vi "Test.vi"() -> ()   [LabVIEW 2014]
uses:
  TypeDefs/TriangleFace.ctl
  TypeDefs/Point3D.ctl
  C:/Users/guss2/Documents/CodeBlocksTest/DLL/bin/Debug/DLL.dll
panel:
  in  "zStart":sgl
  in  "List/Poly":bool
  in  "Layer":i32
  out "XY Graph":cluster{cluster{"X":sgl, "Y":sgl}[]}[](graph)
  out "Length":i32
  out "Triangles":T1[](array[typedef])
  in  "STL Path":path=path "D:/Data/Git/LVslicer/STL2/cone.stl"
  out "NumIntersect":i64
  out "edgeLen":i32[](array[numeric])
  out "List":T3(array[cluster])
  in  "Thick":sgl=0.321
  in  "NumSlices":i32=3
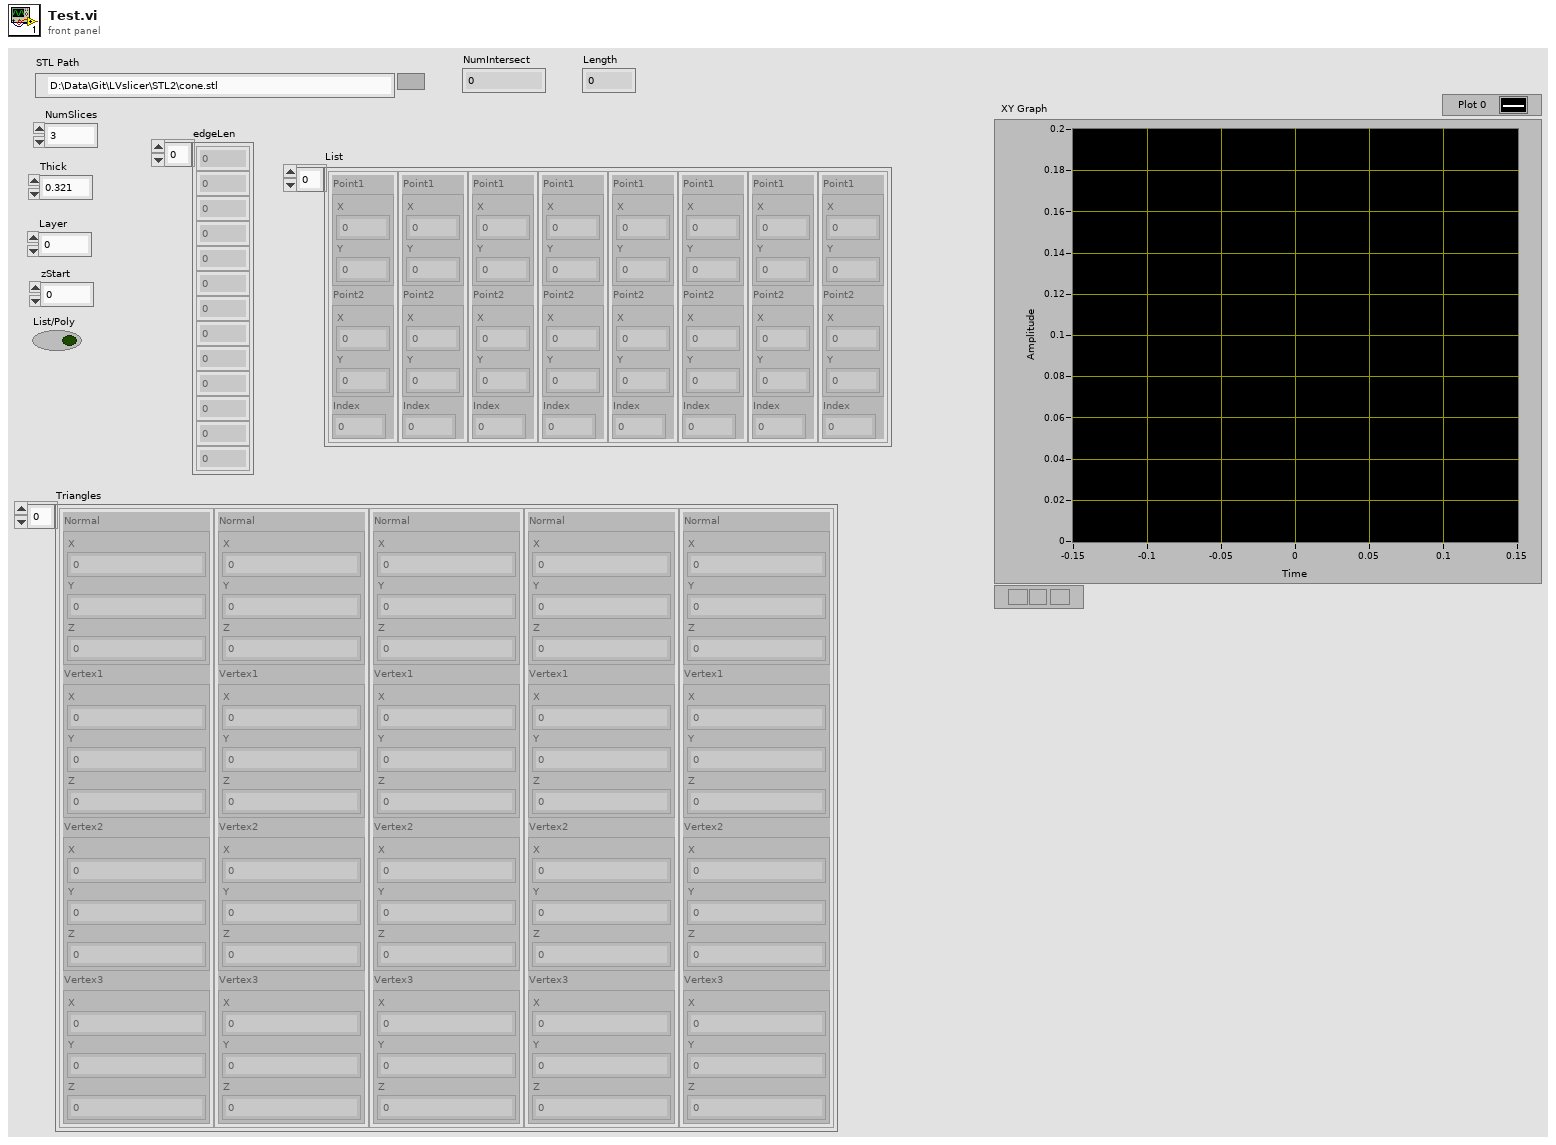
[diagram p1: front panel]
types:
  T1 = typedef "TriangleFace.ctl" = cluster{"Normal":T2, "Vertex1":T2, "Vertex2":T2, "Vertex3":T2}
  T2 = typedef "Point3D.ctl" = cluster{"X":sgl, "Y":sgl, "Z":sgl}
  T3 = cluster{"Point1":cluster{"X":sgl, "Y":sgl}, "Point2":cluster{"X":sgl, "Y":sgl}, "Index":i32}[]
  T4 = cluster{"Point1":cluster{"X":sgl, "Y":sgl}, "Point2":cluster{"X":sgl, "Y":sgl}, "Index":i32}
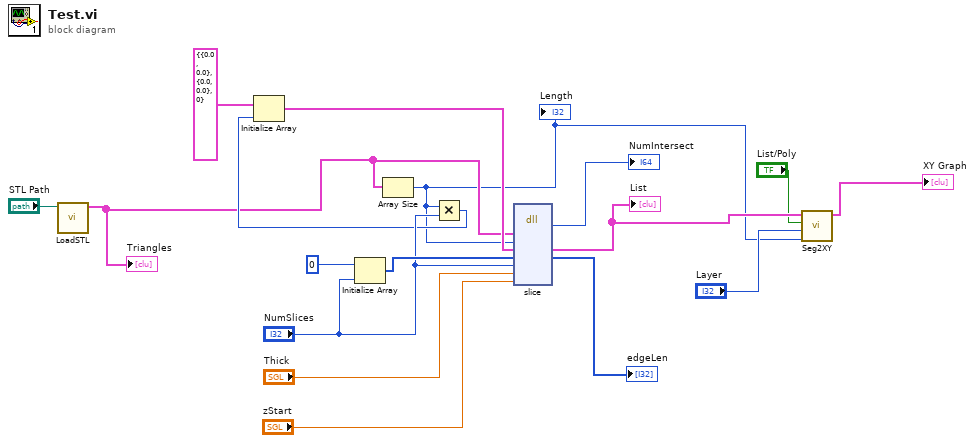
[diagram p0: block diagram]
diagram:
  n1 = call "LoadSTL.vi"("STL Path"="STL Path") -> ("Triangles"=w7:T1[])  [unwired: 8 in, 2 out]
  "Triangles" <- w7
  n2 = Initialize Array(0, "NumSlices") -> (w15:i32[])
  n3 = Array Size(array=w7) -> (size(s)=w4:i32)
  "Length" <- w4
  n4 = Multiply(x=w4, y="NumSlices") -> (x*y=w10:i32)
  n5 = Initialize Array(T4 {"Point1"={"X"=0.0, "Y"=0.0}, "Point2"={"X"=0.0, "Y"=0.0}, "Index"=0} ("Edge"), w10) -> (w9:T3)
  n6 = dll-call lib="C:/Users/guss2/Documents/CodeBlocksTest/DLL/bin/Debug/DLL.dll" fn="slice"("tri"=w7, "length"=w4, "el"=w9, "edgeLen"=w15, "slices"="NumSlices", "thickness"="Thick", "zStart"="zStart") -> ("return type"=→"NumIntersect":i32, "el"=w5:T3, "edgeLen"=→"edgeLen":i32[])  [unwired: 8 in, 2 out]
  "List" <- w5
  n7 = call "Seg2XY.vi"("Length"=w4, "Layer"="Layer", "List/Poly"="List/Poly", "List"=w5) -> ("XY Graph"=→"XY Graph":cluster{cluster{"X":sgl, "Y":sgl}[]}[])  [unwired: 7 in]
